vi "upload.vi"(8 "error in":errorcluster, 9 "timeout per chunk (ms)":i32=300000, 10 "File":path, 11 "Nominal Client in":refnum<class "Nominal Client.lvclass">) -> (0 "error out":errorcluster, 2 "Path to S3 File":string, 3 "Nominal Client out":refnum<class "Nominal Client.lvclass">)   [LabVIEW 2020, in "Nominal Client.lvclass"]
doc: "Uploads a file to Nominal by taking the file path as input and automatically selecting the appropriate upload technique based on the file size. Small files are uploaded in a single operation, while large files are uploaded using a multipart strategy for efficiency and reliability."
uses:
  Nominal Client.lvclass
  Nominal Client.lvclass/Nominal Client.ctl
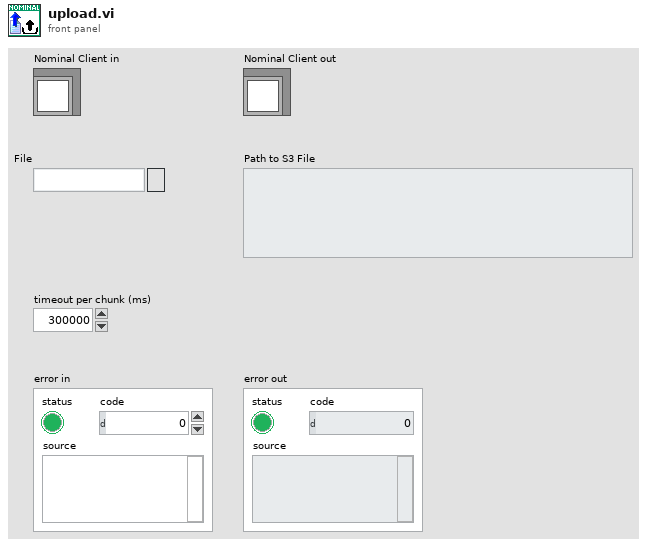
[diagram p1: front panel]
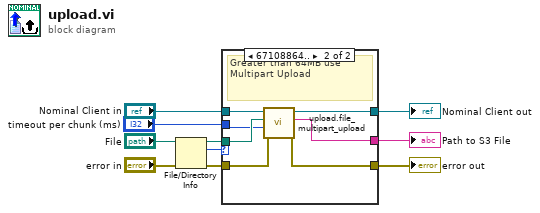
[diagram p0: block diagram]
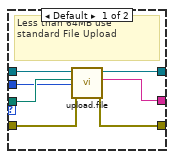
[diagram p2: hidden frame]
diagram:
  n1 = File/Directory Info(path="File", error in="error in") -> (path out=w7:path, size=w9:i64, error out=w4:errorcluster)  [unwired: 4 out]
  n2 = case shown="67108864.." w9 {
    tunnel: w7 -> [w17 w21]
    tunnel: "Nominal Client in" -> [w16 w24]
    tunnel: [w15 w23] -> w5
    tunnel: w4 -> [w14 w20]
    tunnel: [w13 w19] -> w3
    tunnel: [w12 w22] -> w2
    tunnel: "timeout per chunk (ms)" -> [w11 w18]
    frame Default {
      # "Less than 64MB use standard File Upload"
      n3 = call "upload.file.vi"("error in"=w14, "timeout (ms)"=w11, "File"=w17, "Nominal Client in"=w16) -> ("error out"=w13:errorcluster, "Path to S3 File"=w12:string, "Nominal Client out"=w15:refnum<class "Nominal Client.lvclass">)  [unwired: 5 in]
    }
    frame 67108864.. {
      # "Greater than 64MB use Multipart Upload"
      n4 = call "upload.file_multipart_upload.vi"("error in"=w20, "timeout per chunk (ms)"=w18, "File Path"=w21, "Nominal Client in"=w24) -> ("error out"=w19:errorcluster, "S3 Path to File"=w22:string, "Nominal Client out"=w23:refnum<class "Nominal Client.lvclass">)  [unwired: 5 in]
    }
  }
  "Nominal Client out" <- w5
  "error out" <- w3
  "Path to S3 File" <- w2
